vi "Library Name.vi"() -> (3 "library name":string)   [LabVIEW 2017, in "UDP Transceiver.lvclass"]
uses:
  UDP Transceiver.lvclass
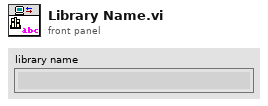
[diagram p1: front panel]
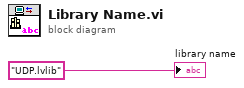
[diagram p0: block diagram]
diagram:
  "library name" <- "UDP.lvlib" ("base error code")
